vi "Read Single Data Point.vi"(8 "error in (no error)":errorcluster, 11 "34401 in":refnum<class "34401.lvclass">) -> (0 "error out":errorcluster, 2 "Value":dbl, 3 "34401 out":refnum<class "34401.lvclass">)   [LabVIEW 2018, in "34401.lvlib" / "34401.lvclass"]
uses:
  34401.lvclass
  34401.lvclass/34401.ctl
  <instrlib>/Agilent 34401/Public/Data/Read (Single Point).vi
  <instrlib>/Agilent 34401/Agilent 34401.lvlib
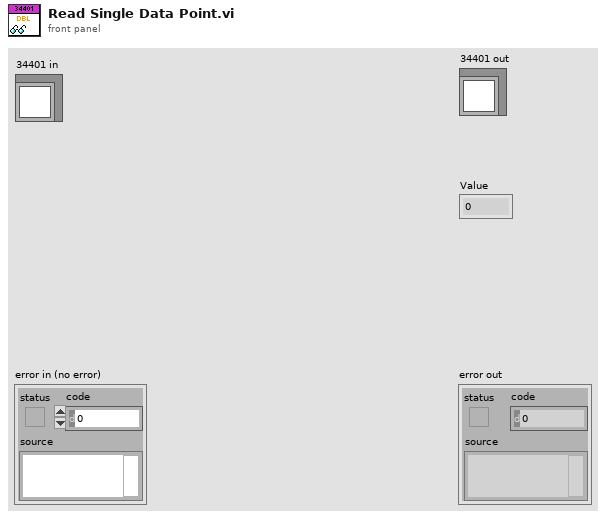
[diagram p1: front panel]
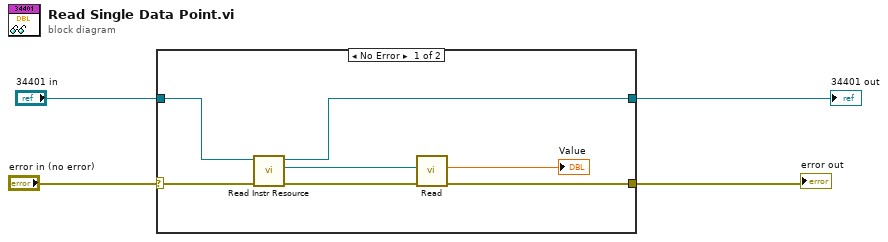
[diagram p0: block diagram]
diagram:
  n1 = case shown="No Error" "error in (no error)" {
    selector: "error in (no error)" -> [w11 w12]
    tunnel: "34401 in" -> [w10 w13]
    tunnel: [w6 w12] -> w2
    tunnel: [w5 w13] -> w1
    frame No Error {
      n2 = call "Read Instr Resource.vi"("error in (no error)"=w11, "34401 in"=w10) -> ("error out"=w9:errorcluster, "Instr Resource"=w8:refnum<visa-resource-name>, "34401 out"=w5:refnum<class "34401.lvclass">)  [unwired: 7 in]
      n3 = call-poly <instrlib>:"Read.vi"("error in (no error)"=w9, "VISA resource name"=w8) -> ("error out"=w6:errorcluster, "Measurement"=→"Value":dbl)  [unwired: 7 in, 1 out]
    }
    frame Error {
    }
  }
  "error out" <- w2
  "34401 out" <- w1
